vi "P100.vi"(11 "Numeric":dbl) -> (3 "PT100":dbl)   [LabVIEW 2017]
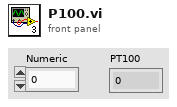
[diagram p1: front panel]
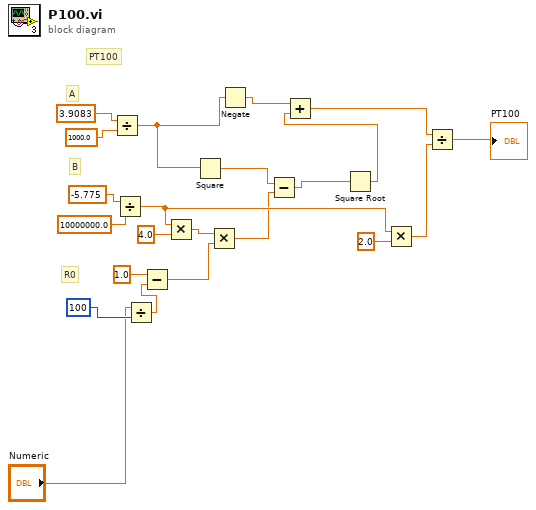
[diagram p0: block diagram]
diagram:
  # "R0"
  # "B"
  # "A"
  # "PT100"
  n1 = Divide(x=3.9083, y=1000.0) -> (x/y=w7:dbl)
  n2 = Divide(x=-5.775, y=10000000.0) -> (x/y=w20:dbl)
  n3 = Divide(x="Numeric", y=100) -> (x/y=w12:dbl)
  n4 = Subtract(x=1.0, y=w12) -> (x-y=w14:dbl)
  n5 = Multiply(x=w20, y=4.0) -> (x*y=w10:dbl)
  n6 = Square(x=w7) -> (x^2=w8:dbl)
  n7 = Multiply(x=w10, y=w14) -> (x*y=w15:dbl)
  n8 = Negate(x=w7) -> (-x=w6:dbl)
  n9 = Subtract(x=w8, y=w15) -> (x-y=w16:dbl)
  n10 = Square Root(x=w16) -> (sqrt(x)=w17:dbl)
  n11 = Add(x=w6, y=w17) -> (x+y=w18:dbl)
  n12 = Multiply(x=w20, y=2.0) -> (x*y=w21:dbl)
  n13 = Divide(x=w18, y=w21) -> (x/y=→"PT100":dbl)
